vi "asset.update_cache.vi"(8 "error in":errorcluster, 11 "asset in":refnum<class "asset.lvclass">) -> (0 "error out":errorcluster, 3 "asset out":refnum<class "asset.lvclass">)   [LabVIEW 2020, in "asset.lvclass"]
uses:
  asset.lvclass
  asset.lvclass/asset.ctl
  <vilib>/JDP Science/JSONtext/Variant to JSON Text.vi
  <vilib>/JDP Science/JSONtext/LVClass Serializer/JSONtext LVClass Serializer.lvclass
  Nominal Client/Nominal Client.lvclass
  Nominal Client/asset.get.vi
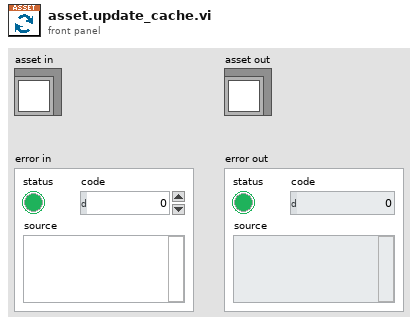
[diagram p1: front panel]
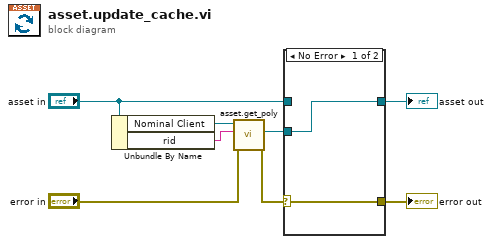
[diagram p0: block diagram]
diagram:
  n1 = Unbundle By Name("asset in") -> ("Nominal Client"=w7:refnum<class "Nominal Client.lvclass">, "rid"=w6:string)
  n2 = call-poly "asset.get_poly.vi"("error in"="error in", "Asset RID"=w6, "Nominal Client in"=w7) -> ("error out"=w4:errorcluster, "Asset"=w1:refnum<class "asset.lvclass">)  [unwired: 6 in, 1 out]
  n3 = case shown="No Error" w4 {
    selector: w4 -> [w9 w12]
    tunnel: [w9 w12] -> w8
    tunnel: [w10 w11] -> w3
    tunnel: "asset in" -> [_ w11]
    tunnel: w1 -> [w10 _]
    frame No Error {
    }
    frame Error {
    }
  }
  "asset out" <- w3
  "error out" <- w8
